vi "Set Visibility.vi"(8 "error in":errorcluster, 11 "DIG_IO in":refnum<class "DIG_IO.lvclass">) -> (0 "error out":errorcluster, 3 "DIG_IO out":refnum<class "DIG_IO.lvclass">)   [LabVIEW 2019, in "DIG_IO.lvlib" / "DIG_IO.lvclass"]
doc: "This routine determines whether the DIO module called is a digital input, or a digital output, and how many Input or output controls to display."
uses:
  Library/DIG_IO.lvclass
  Library/DIG_IO.lvclass/DIG_IO.ctl
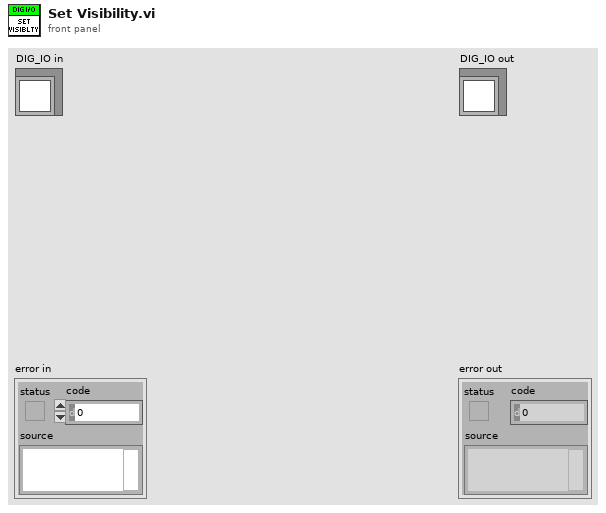
[diagram p1: front panel]
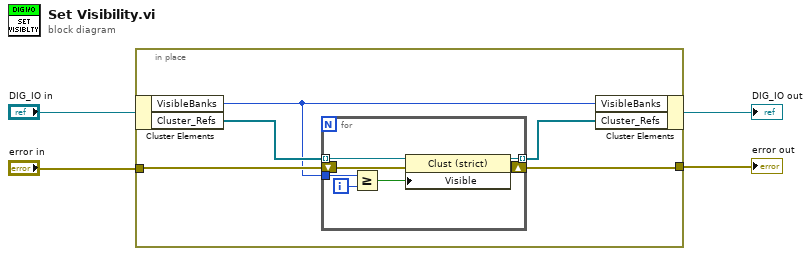
[diagram p0: block diagram]
diagram:
  n1 = in-place {
    in-place-border: "error in" -> [w9]
    in-place-border: [w8] -> w3
    n2 = in-place-cluster #1("DIG_IO in") -> ("VisibleBanks"=w5:u8, "Cluster_Refs"=w7:refnum<vi>[])
    n3 = for {
      shift-right: [w15] -> w8
      shift-left: w9 -> [w16]
      tunnel: w7 -> [w14] mode=indexing
      tunnel: [w13] -> w6 mode=indexing
      tunnel: w5 -> [w11]
      i -> [w12]
      n4 = Greater Or Equal?(x=w11, y=w12) -> (x >= y?=w10:bool)
      n5 = property class="Clust (strict)"(reference=w14, error in=w16, "Visible"=w10) -> (reference out=w13:refnum<vi>, error out=w15:errorcluster)
    }
    n6 = in-place-cluster #1("VisibleBanks"=w5, "Cluster_Refs"=w6) -> (→"DIG_IO out":refnum<class "DIG_IO.lvclass">)
  }
  "error out" <- w3
